vi "Release.vi"(8 "error in (no error)":errorcluster, 11 "Session in":refnum<class "Session.lvclass">) -> (0 "error out":errorcluster)   [LabVIEW 2025, in "CTI.lvlib" / "Session.lvclass"]
doc: "Cleans up all resources and memory managed by the session. This should be called for every session that has been initialized."
uses:
  Session.lvclass
  Session.lvclass/Session.ctl
  DeviceComms/DeviceComms.lvclass
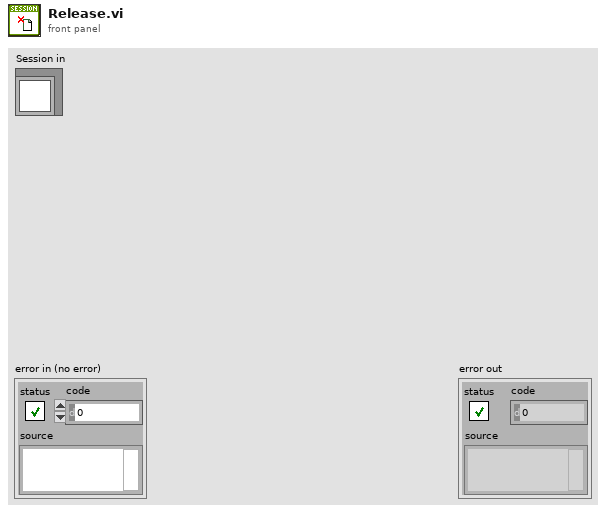
[diagram p1: front panel]
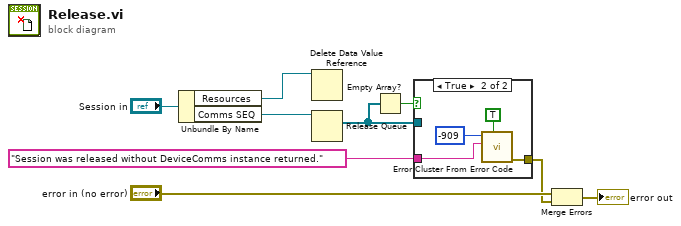
[diagram p0: block diagram]
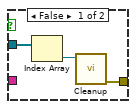
[diagram p2: hidden frame]
diagram:
  n1 = Unbundle By Name("Session in") -> ("Resources"=w1:refnum<data-value>, "Comms SEQ"=w7:refnum<queue>)
  n2 = Delete Data Value Reference(data value reference=w1) -> ()  [unwired: 1 in, 2 out]
  n3 = Release Queue(queue=w7) -> (remaining elements=w6:refnum<class "DeviceComms.lvclass">[])  [unwired: 2 in, 2 out]
  n4 = Empty Array?(array=w6) -> (empty?=w5:bool)
  n5 = case shown="True" w5 {
    tunnel: w6 -> [w12 _]
    tunnel: [w10 w16] -> w2
    tunnel: "Session was released without DeviceComms instance returned." -> [_ w13]
    frame False {
      n6 = Index Array(array=w12) -> (element=w11:refnum<class "DeviceComms.lvclass">)  [unwired: 1 in]
      n7 = call-dynamic "Cleanup.vi"("DeviceComms in"=w11) -> ("error out"=w10:errorcluster)  [unwired: 10 in]
    }
    frame True {
      n8 = call <vilib>:"Error Cluster From Error Code.vi"("show call chain? (False)"=TRUE, "error message (\"\")"=w13, "error code (0)"=-909) -> ("error out"=w16:errorcluster)  [unwired: 6 in]
    }
  }
  n9 = Merge Errors("error in (no error)", w2) -> (→"error out":errorcluster)
